vi "Create HW Defaults.vi"(8 "error in (no error)":errorcluster) -> (0 "error out":errorcluster, 3 "HW out":refnum<class "Process Settings.lvclass">)   [LabVIEW 2017, in "Process Settings.lvclass"]
uses:
  Process Settings.lvclass
  Hardware Settings/Hardware Settings.lvclass
  Type Defs/Process Step Description.ctl
  Type Defs/Item.ctl
  Type Defs/Units.ctl
  Hardware Settings/Type Defs/Hardware Types.ctl
  Hardware Settings/Hardware Types/Generic/Type Defs/Owning System.ctl
  Hardware Settings/Hardware Types/Simulated/Simulated HW.lvclass
  C:/Microcellular Plastics Lab/Hardware Settings/Hardware Types/Generic/Generic Hardware.lvclass
  Hardware Settings/Hardware Types/Generic/Generic Hardware.lvclass/Generic Hardware.ctl
  Hardware Settings/Hardware Settings.lvclass/Hardware Settings.ctl
  Process Settings.lvclass/Process Settings.ctl
  Hardware Settings/Hardware Types/Generic/Accessors/Write Owning System.vi
  Hardware Settings/Hardware Types/Generic/Accessors/Write Description.vi
  Hardware Settings/Accessors/Write Active Channels.vi
  Accessors/Write Hardware Settings.vi
  Accessors/Write Author.vi
  Accessors/Write Filename.vi
  Accessors/Write Time Stamp.vi
  Accessors/Write Process Step Configs.vi
  Hardware Settings/Hardware Types/DAQmx AI/DAQmx AI.lvclass
  Hardware Settings/Hardware Types/DAQmx AO/DAQmx AO.lvclass
  Hardware Settings/Hardware Types/DAQmx DIO/DAQmx DIO.lvclass
  Hardware Settings/Hardware Types/Generic/Generic Hardware.lvclass
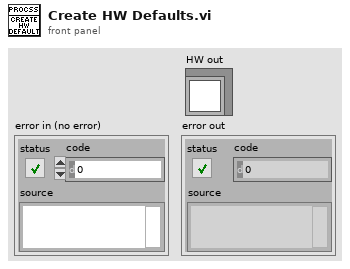
[diagram p1: front panel]
types:
  T1 = typedef "Process Settings.lvclass/Process Step Description.ctl" = cluster{"Item":T2, "Value":dbl, "Units":T3}
  T2 = typedef "Process Settings.lvclass/Item.ctl" = enum16{"", "sheet temperature setpoint", "sheet heating time", "temp element setpoint", "chamber pressure setpoint", "saturation time", "chamber pressure valve setpoint"}
  T3 = typedef "Process Settings.lvclass/Units.ctl" = enum16{"°F", "°C", "Seconds", "Minutes", "PSIA", "V"}
  T4 = typedef "Hardware Settings.lvclass/Hardware Types.ctl" = enum16{"Tank Chamber Pressure and Temperature", "Tank Valve Controls", "Motor On/Off and Direction Control", "Limit Switches", "IR Temperature", "Pneumatic Cylinder Actuation", "Expansion Temperature Setpoint"}
  T5 = typedef "Generic Hardware.lvclass/Owning System.ctl" = enum16{"Saturation", "Expansion"}
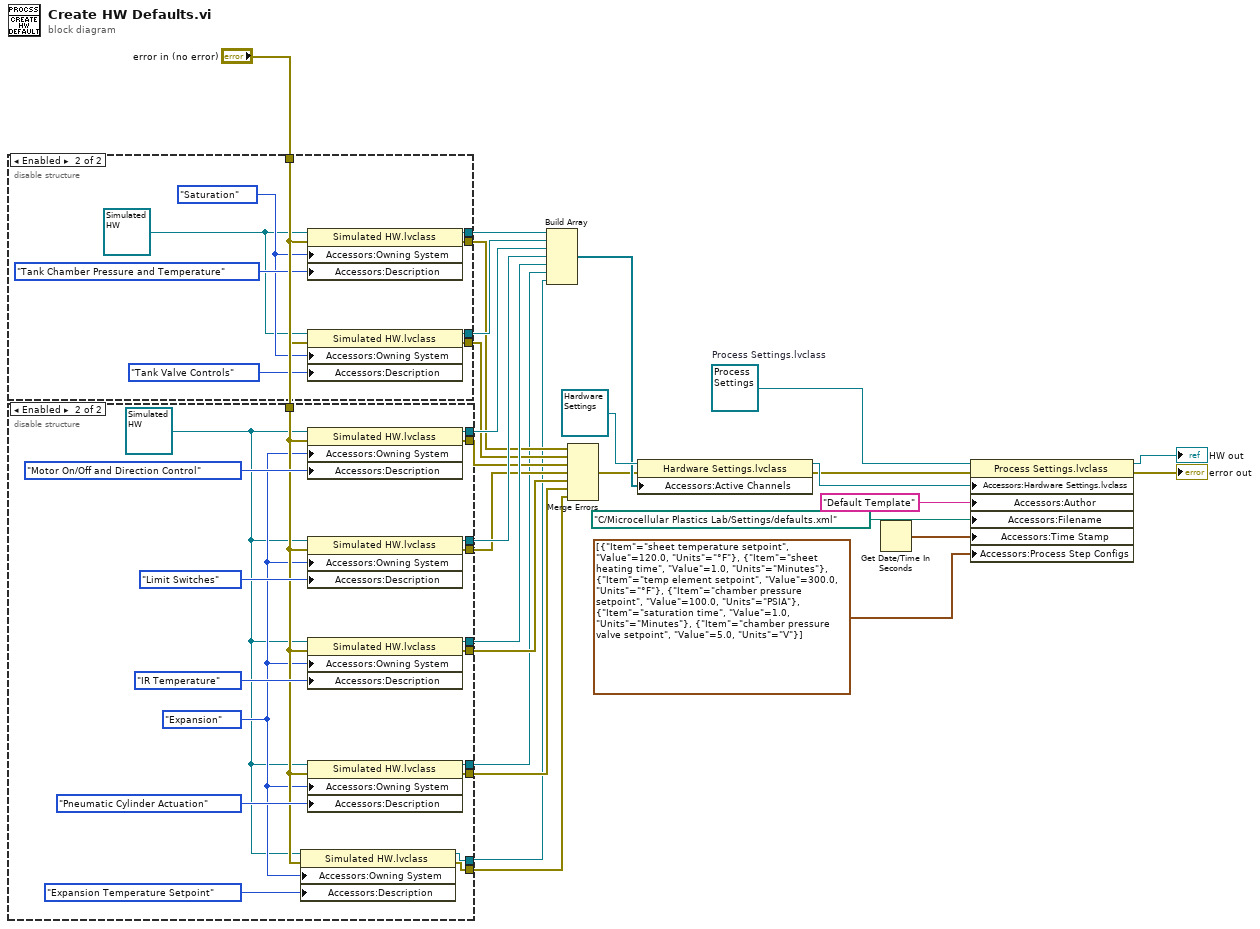
[diagram p0: block diagram]
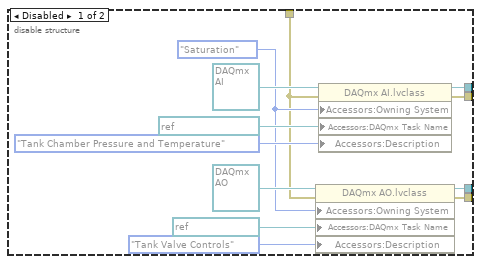
[diagram p2: hidden frame]
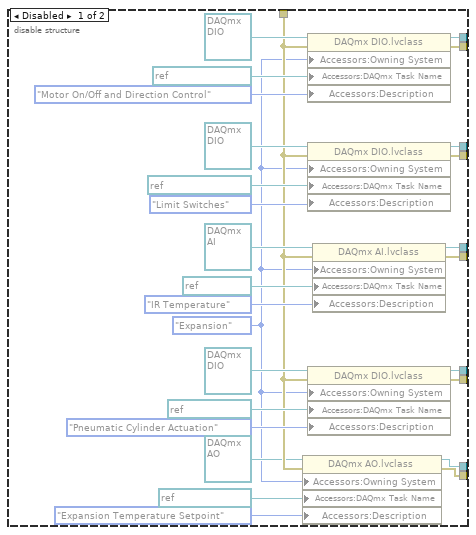
[diagram p3: hidden frame]
diagram:
  w9 = refnum<class "Process Settings.lvclass"> refnum  # Process Settings.lvclass
  n1 = disable-structure shown="Enabled" {
    disable-tunnel: [w37 w48] -> w26
    disable-tunnel: [w36 w47] -> w23
    disable-tunnel: [w31 w44] -> w20
    disable-tunnel: [w30 w43] -> w19
    disable-tunnel: "error in (no error)" -> [w28 w41]
    frame Disabled {
      w29 = Owning_System."Saturation" ("Owning System")
      n2 = property class="DAQmx AO.lvclass"(reference=refnum<class "DAQmx AO.lvclass"> refnum ("DAQmx AO.lvclass"), error in=w28, "Accessors:Owning System"=w29, "Accessors:DAQmx Task Name"=refnum<k21> "SatValveCtl" ("DAQmx Task Name"), "Accessors:Description"=Hardware_Types."Tank Valve Controls") -> (reference out=w36:refnum<class "DAQmx AO.lvclass">, error out=w30:errorcluster)
      n3 = property class="DAQmx AI.lvclass"(reference=refnum<class "DAQmx AI.lvclass"> refnum ("DAQmx AI.lvclass"), error in=w28, "Accessors:Owning System"=w29, "Accessors:DAQmx Task Name"=refnum<k21> "SatTankTemp" ("DAQmx Task Name"), "Accessors:Description"=Hardware_Types."Tank Chamber Pressure and Temperature") -> (reference out=w37:refnum<class "DAQmx AI.lvclass">, error out=w31:errorcluster)
    }
    frame Enabled {
      w40 = refnum<class "Simulated HW.lvclass"> refnum ("Simulated HW.lvclass")
      w42 = Owning_System."Saturation" ("Owning System")
      n4 = property class="Simulated HW.lvclass"(reference=w40, error in=w41, "Accessors:Owning System"=w42, "Accessors:Description"=Hardware_Types."Tank Chamber Pressure and Temperature") -> (reference out=w48:refnum<class "Simulated HW.lvclass">, error out=w44:errorcluster)
      n5 = property class="Simulated HW.lvclass"(reference=w40, error in=w41, "Accessors:Owning System"=w42, "Accessors:Description"=Hardware_Types."Tank Valve Controls") -> (reference out=w47:refnum<class "Simulated HW.lvclass">, error out=w43:errorcluster)
    }
  }
  n6 = disable-structure shown="Enabled" {
    disable-tunnel: [w74 w93] -> w25
    disable-tunnel: [w65 w89] -> w22
    disable-tunnel: [w64 w88] -> w21
    disable-tunnel: [w63 w87] -> w18
    disable-tunnel: [w62 w86] -> w17
    disable-tunnel: [w61 w85] -> w16
    disable-tunnel: "error in (no error)" -> [w53 w79]
    disable-tunnel: [w57 w83] -> w13
    disable-tunnel: [w56 w82] -> w12
    disable-tunnel: [w54 w80] -> w11
    disable-tunnel: [w49 w77] -> w10
    frame Disabled {
      w51 = Owning_System."Expansion" ("Owning System")
      n7 = property class="DAQmx AO.lvclass"(reference=refnum<class "DAQmx AO.lvclass"> refnum ("DAQmx AO.lvclass"), error in=w53, "Accessors:Owning System"=w51, "Accessors:DAQmx Task Name"=refnum<k21> "ExpTempSet" ("DAQmx Task Name"), "Accessors:Description"=Hardware_Types."Expansion Temperature Setpoint" ("Description")) -> (reference out=w49:refnum<class "DAQmx AO.lvclass">, error out=w54:errorcluster)
      n8 = property class="DAQmx DIO.lvclass"(reference=refnum<class "DAQmx DIO.lvclass"> refnum ("DAQmx DIO.lvclass"), error in=w53, "Accessors:Owning System"=w51, "Accessors:DAQmx Task Name"=refnum<k21> "MotorOn_Off" ("DAQmx Task Name"), "Accessors:Description"=Hardware_Types."Motor On/Off and Direction Control" ("Description")) -> (reference out=w74:refnum<class "DAQmx DIO.lvclass">, error out=w63:errorcluster)
      n9 = property class="DAQmx DIO.lvclass"(reference=refnum<class "DAQmx DIO.lvclass"> refnum ("DAQmx DIO.lvclass"), error in=w53, "Accessors:Owning System"=w51, "Accessors:DAQmx Task Name"=refnum<k21> "Limit Switches" ("DAQmx Task Name"), "Accessors:Description"=Hardware_Types."Limit Switches" ("Description")) -> (reference out=w65:refnum<class "DAQmx DIO.lvclass">, error out=w62:errorcluster)
      n10 = property class="DAQmx DIO.lvclass"(reference=refnum<class "DAQmx DIO.lvclass"> refnum ("DAQmx DIO.lvclass"), error in=w53, "Accessors:Owning System"=w51, "Accessors:DAQmx Task Name"=refnum<k21> "PneumAct" ("DAQmx Task Name"), "Accessors:Description"=Hardware_Types."Pneumatic Cylinder Actuation" ("Description")) -> (reference out=w56:refnum<class "DAQmx DIO.lvclass">, error out=w57:errorcluster)
      n11 = property class="DAQmx AI.lvclass"(reference=refnum<class "DAQmx AI.lvclass"> refnum ("DAQmx AI.lvclass"), error in=w53, "Accessors:Owning System"=w51, "Accessors:DAQmx Task Name"=refnum<k21> "IRTemp" ("DAQmx Task Name"), "Accessors:Description"=Hardware_Types."IR Temperature" ("Description")) -> (reference out=w64:refnum<class "DAQmx AI.lvclass">, error out=w61:errorcluster)
    }
    frame Enabled {
      w76 = refnum<class "Simulated HW.lvclass"> refnum ("Simulated HW.lvclass")
      w78 = Owning_System."Expansion" ("Owning System")
      n12 = property class="Simulated HW.lvclass"(reference=w76, error in=w79, "Accessors:Owning System"=w78, "Accessors:Description"=Hardware_Types."Expansion Temperature Setpoint" ("Description")) -> (reference out=w77:refnum<class "Simulated HW.lvclass">, error out=w80:errorcluster)
      n13 = property class="Simulated HW.lvclass"(reference=w76, error in=w79, "Accessors:Owning System"=w78, "Accessors:Description"=Hardware_Types."Motor On/Off and Direction Control" ("Description")) -> (reference out=w93:refnum<class "Simulated HW.lvclass">, error out=w87:errorcluster)
      n14 = property class="Simulated HW.lvclass"(reference=w76, error in=w79, "Accessors:Owning System"=w78, "Accessors:Description"=Hardware_Types."Limit Switches" ("Description")) -> (reference out=w89:refnum<class "Simulated HW.lvclass">, error out=w86:errorcluster)
      n15 = property class="Simulated HW.lvclass"(reference=w76, error in=w79, "Accessors:Owning System"=w78, "Accessors:Description"=Hardware_Types."IR Temperature" ("Description")) -> (reference out=w88:refnum<class "Simulated HW.lvclass">, error out=w85:errorcluster)
      n16 = property class="Simulated HW.lvclass"(reference=w76, error in=w79, "Accessors:Owning System"=w78, "Accessors:Description"=Hardware_Types."Pneumatic Cylinder Actuation" ("Description")) -> (reference out=w82:refnum<class "Simulated HW.lvclass">, error out=w83:errorcluster)
    }
  }
  n17 = Build Array(w26, w23, w25, w22, w21, w12, w10) -> (w24:refnum<class "Simulated HW.lvclass">[])
  n18 = Merge Errors(w20, w19, w18, w17, w16, w13, w11) -> (w15:errorcluster)
  n19 = property class="Hardware Settings.lvclass"(reference=refnum<class "Hardware Settings.lvclass"> refnum ("Hardware Settings.lvclass"), error in=w15, "Accessors:Active Channels"=w24) -> (reference out=w8:refnum<class "Hardware Settings.lvclass">, error out=w5:errorcluster)
  n20 = Get Date/Time In Seconds() -> (seconds since 1Jan1904=w2:timestamp)
  n21 = property class="Process Settings.lvclass"(reference=w9, error in=w5, "Accessors:Hardware Settings.lvclass"=w8, "Accessors:Author"="Default Template" ("Author"), "Accessors:Filename"=path "C:/Microcellular Plastics Lab/Settings/defaults.xml" ("Filename"), "Accessors:Time Stamp"=w2, "Accessors:Process Step Configs"=T1[] [{"Item"=enum."sheet temperature setpoint", "Value"=120.0, "Units"=enum."°F"}, {"Item"=enum."sheet heating time", "Value"=1.0, "Units"=enum."Minutes"}, {"Item"=enum."temp element setpoint", "Value"=300.0, "Units"=enum."°F"}, {"Item"=enum."chamber pressure setpoint", "Value"=100.0, "Units"=enum."PSIA"}, {"Item"=enum."saturation time", "Value"=1.0, "Units"=enum."Minutes"}, {"Item"=enum."chamber pressure valve setpoint", "Value"=5.0, "Units"=enum."V"}] ("Process Step Configs")) -> (reference out=→"HW out":refnum<class "Process Settings.lvclass">, error out=→"error out":errorcluster)
